vi "Stage 2.3 myDAQ - Measuring Heartrate.vi"() -> ()   [LabVIEW 2020]
uses:
  <vilib>/measure/matone.llb/Extract Single Tone Information 1 Chan.vi
  <vilib>/measure/NI_MAPro.lvlib
panel:
  in  "Addition signal to remove (0) [s]":dbl
  out "Pulse":dbl
  out "Filtered":waveform(dbl)(graph)
  in  "Samples size (10) [s]":i32=10
  out "error out":errorcluster
  out "Raw":waveform(dbl)(graph)
  in  "Stop":bool
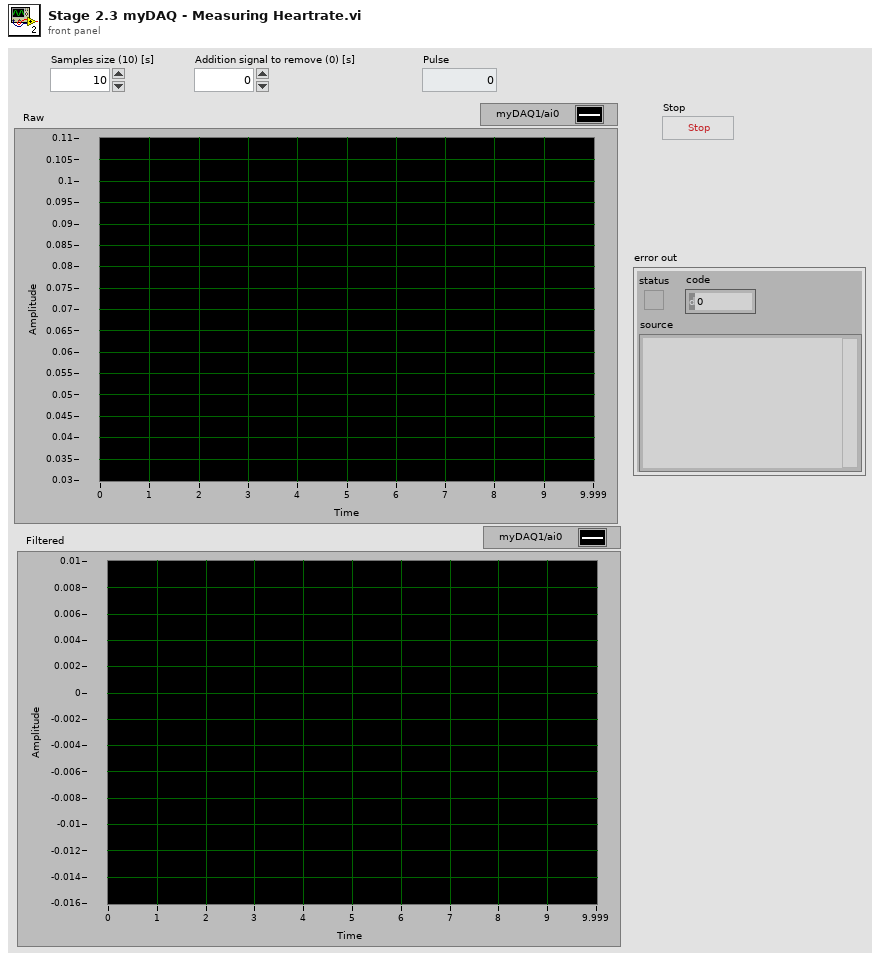
[diagram p1: front panel]
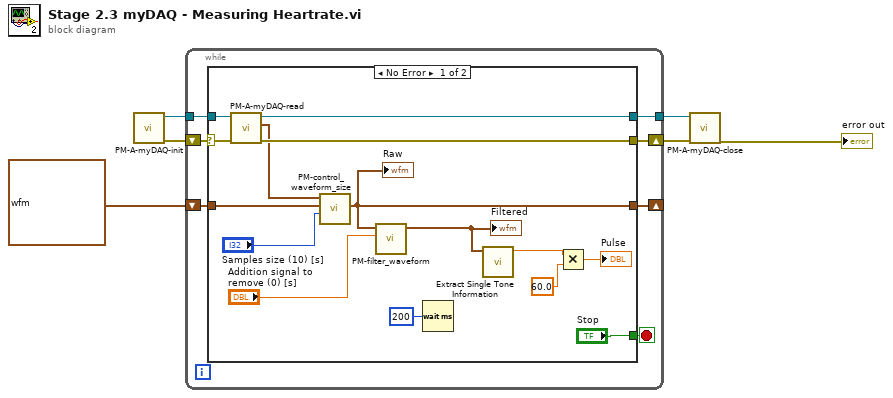
[diagram p0: block diagram]
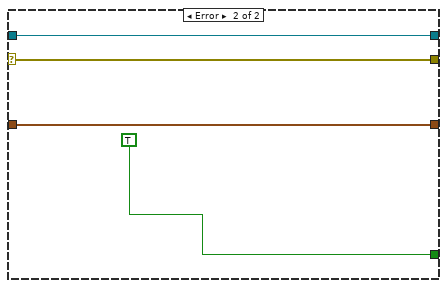
[diagram p2: hidden frame]
diagram:
  n1 = call "PM-A-myDAQ-init.vi"() -> ("error out"=w5:errorcluster, "Refnum out"=w4:refnum<k21>)  [unwired: 10 in]
  n2 = while {
    tunnel: w4 -> [w13]
    tunnel: [w11] -> w3
    shift-right: [w10] -> w2
    shift-left: w5 -> [w12]
    shift-right: [w7] -> _
    shift-left: waveform(dbl) {"t0"=timestamp(0 s since 1904-01-01), "dt"=0.0, "Y"=[]} ("data") -> [w8]
    stop <- w9 stop-if-true
    n3 = case shown="No Error" w12 {
      selector: w12 -> [w27 w31]
      tunnel: w13 -> [w28 w30]
      tunnel: [w25 w30] -> w11
      tunnel: [w24 w31] -> w10
      tunnel: ["Stop" TRUE ("Stop")] -> w9
      tunnel: w8 -> [w21 w29]
      tunnel: [w19 w29] -> w7
      frame No Error {
        n4 = call "PM-A-myDAQ-read.vi"("error in (no error)"=w27, "Refnum in"=w28) -> ("error out"=w24:errorcluster, "data"=w20:waveform(dbl), "Refnum out"=w25:refnum<k21>)  [unwired: 7 in]
        n5 = call "PM-control_waveform_size.vi"("Samples s"="Samples size (10) [s]", "old waveform"=w21, "New waveform"=w20) -> ("waveform"=w19:waveform(dbl))  [unwired: 8 in]
        "Raw" <- w19
        n6 = call "PM-filter_waveform.vi"("Addition signal to remove (0) [s]"="Addition signal to remove (0) [s]", "waveform in"=w19) -> ("waveform out"=w18:waveform(dbl))  [unwired: 8 in, 1 out]
        "Filtered" <- w18
        n7 = Wait (ms)(milliseconds to wait=u32 200) -> ()  [unwired: 1 out]
        n8 = call-poly <vilib>:"Extract Single Tone Information.vi"("time signal in"=w18) -> ("detected frequency"=w17:dbl)  [unwired: 5 in, 5 out]
        n9 = Multiply(x=w17, y=60.0) -> (x*y=→"Pulse":dbl)
      }
      frame Error {
      }
    }
  }
  n10 = call "PM-A-myDAQ-close.vi"("error in (no error)"=w2, "Refnum in"=w3) -> ("error out"=→"error out":errorcluster)  [unwired: 9 in]
